vi "Not Boolean Array (U64).vi"(4 "X":bool[](array[boolean])=[FALSE, FALSE, FALSE, FALSE, FALSE, FALSE, FALSE, TRUE, FALSE, FALSE, FALSE, FALSE, FALSE, FALSE, FALSE, FALSE, FALSE, FALSE, FALSE, FALSE, FALSE, FALSE, FALSE, FALSE, FALSE, FALSE, FALSE, FALSE, FALSE, FALSE, FALSE, FALSE, FALSE, FALSE, FALSE, FALSE, FALSE, FALSE, FALSE, FALSE, FALSE, FALSE, FALSE, FALSE, FALSE, FALSE, FALSE, FALSE, FALSE, FALSE, FALSE, FALSE, FALSE, FALSE, FALSE, FALSE, FALSE, FALSE, FALSE, FALSE, FALSE, FALSE, FALSE, FALSE]) -> (1 "Not X":bool[](array[boolean]))   [LabVIEW 2011]
doc: "This VI performs not operation on Boolean Array of Size 64"
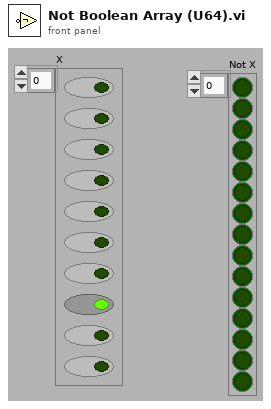
[diagram p1: front panel]
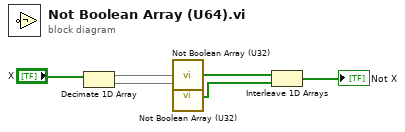
[diagram p0: block diagram]
diagram:
  n1 = Decimate 1D Array("X") -> (w5:bool[], w4:bool[])
  n2 = call <userlib>:"Not Boolean Array (U32).vi"("X"=w5) -> ("Not X"=w2:bool[])  [unwired: 4 in]
  n3 = call <userlib>:"Not Boolean Array (U32).vi"("X"=w4) -> ("Not X"=w3:bool[])  [unwired: 4 in]
  n4 = Interleave 1D Arrays(w2, w3) -> (→"Not X":bool[])
